vi "TurnToDegrees.vi"(4 "Timeout (ms)":u32=2000, 6 "Start time":u32, 7 "Steer PID gains":T1={"proportional gain (Kc)"=0.05, "integral time (Ti, min)"=0.01, "derivative time (Td, min)"=0.002} {"derivative time (Td, min)" format="%#.7g"; "integral time (Ti, min)" format="%#.6g"; "proportional gain (Kc)" format="%#.6g"}, 8 "error in (no error)":errorcluster, 9 "Degrees":dbl, 10 "Steering Saturation":dbl=1.0, 11 "Steer Margin":dbl=3.0) -> (0 "error out":errorcluster, 2 "Done":bool, 3 "RobotDriveDevRef Out":T2={"DevStatus"={"status"=FALSE, "code"=0, "source"=""}, "Motors[]"=[], "Square Inputs"=FALSE, "Max Output"=1.0, "Isochronous"=FALSE})   [LabVIEW 2013]
uses:
  <vilib>/Rock Robotics/WPI/RobotDrive/WPI_RobotDriveDevRef.ctl
  <vilib>/Rock Robotics/WPI/MotorControl/WPI_MotorControlDeviceRef.ctl
  <vilib>/Rock Robotics/SystemInterfaces/Typedef/FPGA_TypedefDigitalModule.ctl
  <vilib>/Rock Robotics/SystemInterfaces/DIO/FPGA_DIOPWMChannel.ctl
  <vilib>/Rock Robotics/WPI/PWM/WPI_PWMDeadband.ctl
  <vilib>/Rock Robotics/WPI/CAN/Jaguar/SubVIs/WPI_CANJaguar_ControlMode.ctl
  <vilib>/Rock Robotics/WPI/PWM/WPI_PWMTransform_ConPane.ctl
  Robot Global Data.vi
  <vilib>/Rock Robotics/WPI/RobotDrive/WPI_RobotDriveGetSetRefNum.vi
  <vilib>/addons/control/pid/NI_PID_pid.lvlib
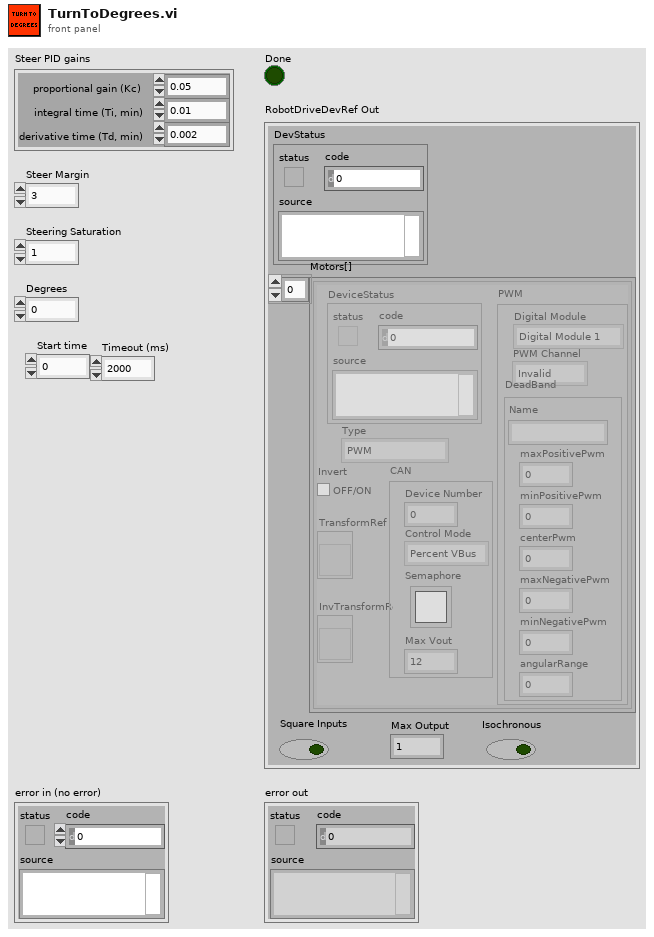
[diagram p1: front panel]
types:
  T1 = cluster{"proportional gain (Kc)":dbl, "integral time (Ti, min)":dbl, "derivative time (Td, min)":dbl}
  T2 = typedef "WPI_RobotDriveDevRef.ctl" = cluster{"DevStatus":errorcluster, "Motors[]":T3[], "Square Inputs":bool, "Max Output":dbl, "Isochronous":bool}
  T3 = typedef "WPI_MotorControlDeviceRef.ctl" = cluster{"DeviceStatus":errorcluster, "Type":enum16{"PWM", "CAN"}, "PWM":cluster{"Digital Module":T4, "PWM Channel":T5, "DeadBand":T6}, "CAN":cluster{"Device Number":u8, "Control Mode":T7, "Semaphore":T8, "Max Vout":dbl}, "Invert":bool, "TransformRef":T9, "InvTransformRef":T9}
  T4 = typedef "FPGA_TypedefDigitalModule.ctl" = enum16{"Digital Module 1", "Digital Module 2"}
  T5 = typedef "FPGA_DIOPWMChannel.ctl" = enum8{"PWM 1", "PWM 2", "PWM 3", "PWM 4", "PWM 5", "PWM 6", "PWM 7", "PWM 8", "PWM 9", "PWM 10", "Invalid"}
  T6 = typedef "WPI_PWMDeadband.ctl" = cluster{"Name":string, "maxPositivePwm":i32, "minPositivePwm":i32, "centerPwm":i32, "maxNegativePwm":i32, "minNegativePwm":i32, "angularRange":u16}
  T7 = typedef "WPI_CANJaguar_ControlMode.ctl" = enum8{"Percent VBus", "Current", "Speed", "Position", "Voltage"}
  T8 = typedef "Semaphore RefNum" = refnum<k1>
  T9 = typedef "WPI_PWMTransform_ConPane.ctl" = refnum<vi>
  T10 = typedef "Position Typedef.ctl" = cluster{"X":dbl, "Y":dbl, "Heading":dbl}
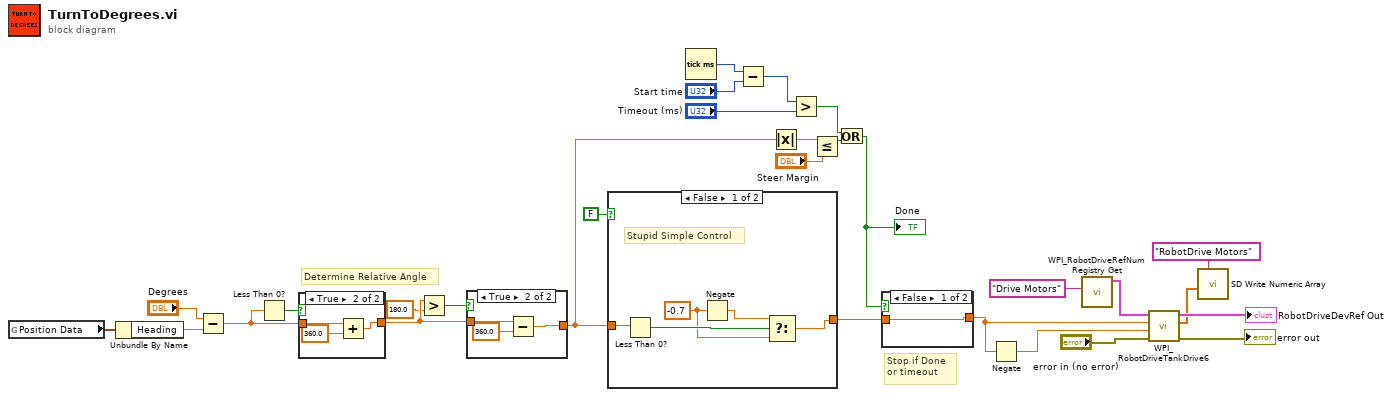
[diagram p0: block diagram]
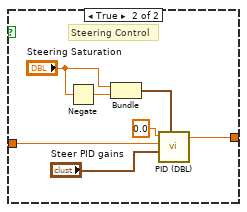
[diagram p2: hidden frame]
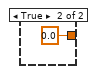
[diagram p3: hidden frame]
diagram:
  # "Stop if Done \nor timeout"
  # "Determine Relative Angle"
  n1 = global read "Robot Global Data.vi" "Position Data"() -> (w18:T10)
  n2 = Unbundle By Name(w18) -> ("Heading"=w19:dbl)
  n3 = Subtract(x="Degrees", y=w19) -> (x-y=w25:dbl)
  n4 = Less Than 0?(x=w25) -> (x < 0?=w23:bool)
  n5 = case shown="True" w23 {
    tunnel: w25 -> [w30 w32]
    tunnel: [w30 w31] -> w24
    frame False {
    }
    frame True {
      n6 = Add(x=w32, y=360.0) -> (x+y=w31:dbl)
    }
  }
  n7 = Greater?(x=w24, y=180.0) -> (0:w22:bool)
  n8 = case shown="True" w22 {
    tunnel: w24 -> [w34 w37]
    tunnel: [w34 w36] -> w2
    frame False {
    }
    frame True {
      n9 = Subtract(x=w37, y=360.0) -> (x-y=w36:dbl)
    }
  }
  n10 = case shown="False" FALSE {
    tunnel: [w40 w49] -> w26
    tunnel: w2 -> [w42 w43]
    frame False {
      w38 = -0.7 ("x")
      # "Stupid Simple Control"
      n11 = Less Than 0?(x=w42) -> (x < 0?=w41:bool)
      n12 = Negate(x=w38) -> (-x=w39:dbl)
      n13 = Select(t=w39, s=w41, f=w38) -> (s? t:f=w40:dbl)
    }
    frame True {
      # "Steering Control"
      n14 = Negate(x="Steering Saturation") -> (-x=w45:dbl)
      n15 = Bundle("Steering Saturation"="Steering Saturation", w45) -> (w46:cluster{"Steering Saturation":dbl, dbl})  [unwired: 1 out]
      n16 = call <vilib>:"PID (DBL).vi"("output range"=w46, "PID gains"="Steer PID gains", "process variable"=w43, "setpoint"=0.0) -> ("output"=w49:dbl)  [unwired: 2 in, 5 out]
    }
  }
  n17 = Tick Count (ms)() -> (millisecond timer value=w9:u32)
  n18 = Subtract(x=w9, y="Start time") -> (x-y=w8:u32)
  n19 = Absolute Value(x=w2) -> (abs(x)=w10:dbl)
  n20 = Greater?(x=w8, y="Timeout (ms)") -> (0:w5:bool)
  n21 = Less Or Equal?(x=w10, y="Steer Margin") -> (x <= y?=w6:bool)
  n22 = Or(x=w5, y=w6) -> (x .or. y?=w4:bool)
  "Done" <- w4
  n23 = case shown="False" w4 {
    tunnel: w26 -> [w50 _]
    tunnel: [w50 0.0 ("output")] -> w27
    frame False {
    }
    frame True {
    }
  }
  n24 = Negate(x=w27) -> (-x=w17:dbl)
  n25 = call <vilib>:"WPI_RobotDriveRefNum Registry Get.vi"("refnum name"="Drive Motors") -> ("RobotDriveDevRef"=w14:T2)  [unwired: 1 in, 9 out]
  n26 = call "WPI_RobotDriveTankDrive6.vi"("error in (no error)"="error in (no error)", "Right axis value"=w17, "Left axis value"=w27, "RobotDriveDevRef"=w14) -> ("error out"=→"error out":errorcluster, "Motor Values"=w16:dbl[], "RobotDriveDevRef"=→"RobotDriveDevRef Out":T2)  [unwired: 5 in]
  n27 = call <vilib>:"SD Write Numeric Array.vi"("Numeric Array"=w16, "Name"="RobotDrive Motors") -> ()  [unwired: 8 in, 2 out]
